vi "GetLogQueue.vi"(8 "error in (no error)":errorcluster) -> (0 "error out":errorcluster, 3 "Queue Out":refnum<queue>)   [LabVIEW 2016, in "Log4Lv.lvlib"]
doc: "Use this template to build a VI to use as a subVI."
uses:
  Log4Lv.lvlib
  Config Global.vi
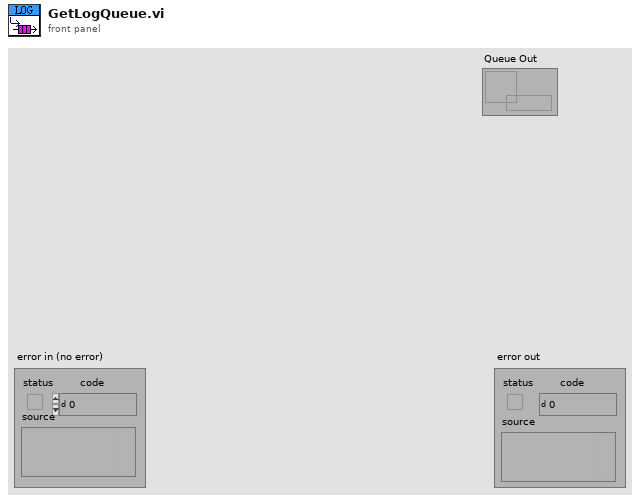
[diagram p1: front panel]
types:
  T1 = cluster{"LogName":string, "Level":enum16{"Disable", "Error", "Warn", "Info", "Debug"}, "LogFolder":path, "MaxFileSize":i32, "FileExtension":string, "TimeSytle":string, "LogStyle":string}
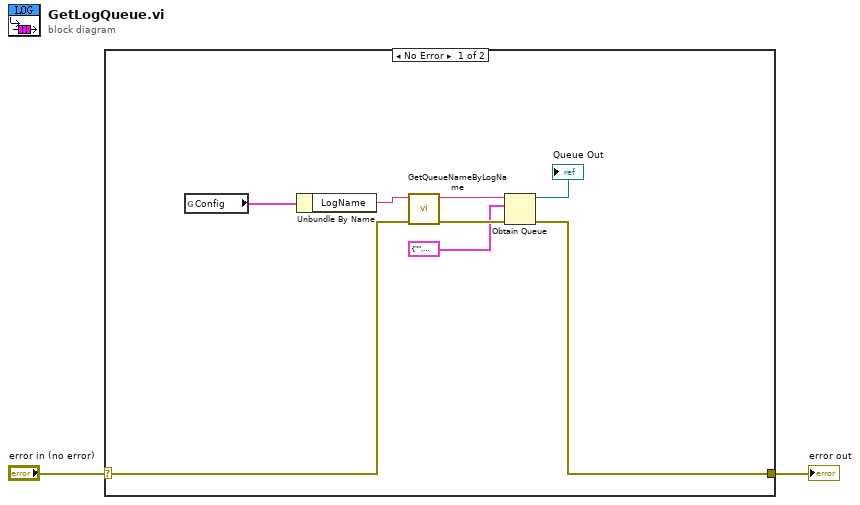
[diagram p0: block diagram]
diagram:
  n1 = case shown="No Error" "error in (no error)" {
    selector: "error in (no error)" -> [w5 w11]
    tunnel: [w4 w11] -> w1
    frame No Error {
      n2 = global read "Config Global.vi" "Config"() -> (w10:T1)
      n3 = Unbundle By Name(w10) -> ("LogName"=w9:string)
      n4 = call "GetQueueNameByLogName.vi"("error in (no error)"=w5, "LogName"=w9) -> ("error out"=w7:errorcluster, "QueueName"=w8:string)  [unwired: 8 in]
      n5 = Obtain Queue(name (unnamed)=w8, element data type=cluster{"Cmd":string, "Data":variant} {"Cmd"="", "Data"=variant}, error in (no error)=w7) -> (queue out=→"Queue Out":refnum<queue>, error out=w4:errorcluster)  [unwired: 2 in, 1 out]
    }
    frame Error {
    }
  }
  "error out" <- w1
